vi "Save Lockin Metadata.vi"(8 "error in (no error)":errorcluster, 11 "Lockin Digitizer Driver in":refnum<class "Lockin Digitizer Driver.lvclass">) -> (0 "error out":errorcluster, 3 "Lockin Digitizer Driver out":refnum<class "Lockin Digitizer Driver.lvclass">)   [LabVIEW 2024, in "Lockin Digitizer Driver.lvclass"]
uses:
  Lockin Digitizer Driver.lvclass
  Pulse Driver.lvclass/Pulse Driver.ctl
  SoftwareLockin/Lockin Parameters.ctl
  Read tdms file.vi
  Write tdms file.vi
  Lockin Digitizer Driver.lvclass/Lockin Digitizer Driver.ctl
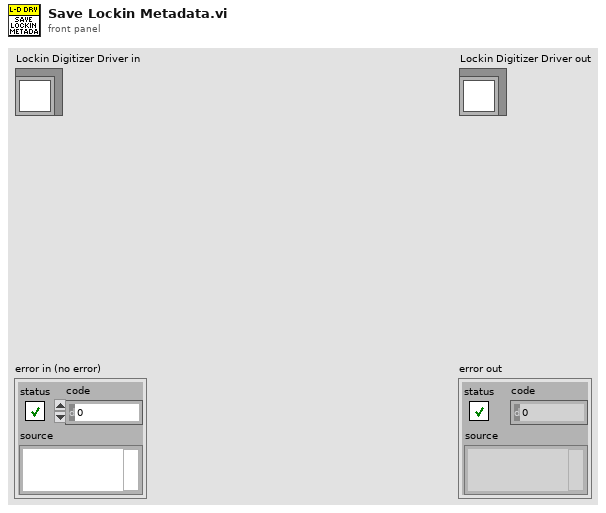
[diagram p1: front panel]
types:
  T1 = typedef "Lockin Digitizer Configuration.ctl" = cluster{"Post-trigger delay":dbl, "Post-trigger duration":dbl, "Rate":dbl, "Ranges":dbl[], "Re-name channels":string[], "Active channels":string, "External\nclock":bool, "Monitor time\nconstant":dbl, "Sync":bool, "Lock-in input channel phases":dbl[], "Output channels configuration":T2[]}
  T2 = typedef "Output Channel Configuration.ctl" = cluster{"Input channels":string, "Frequency":dbl, "Output amplitude":dbl, "Output channel number":i32}
  T3 = typedef "Lockin Parameters.ctl" = cluster{"Frequency":dbl, "Phase":dbl, "Syncronous":bool, "Points per sine wave":i32, "DDS":bool, "Frequency word":u32, "Phase word":u32, "DDS modulus":i64, "DDS clock":dbl}
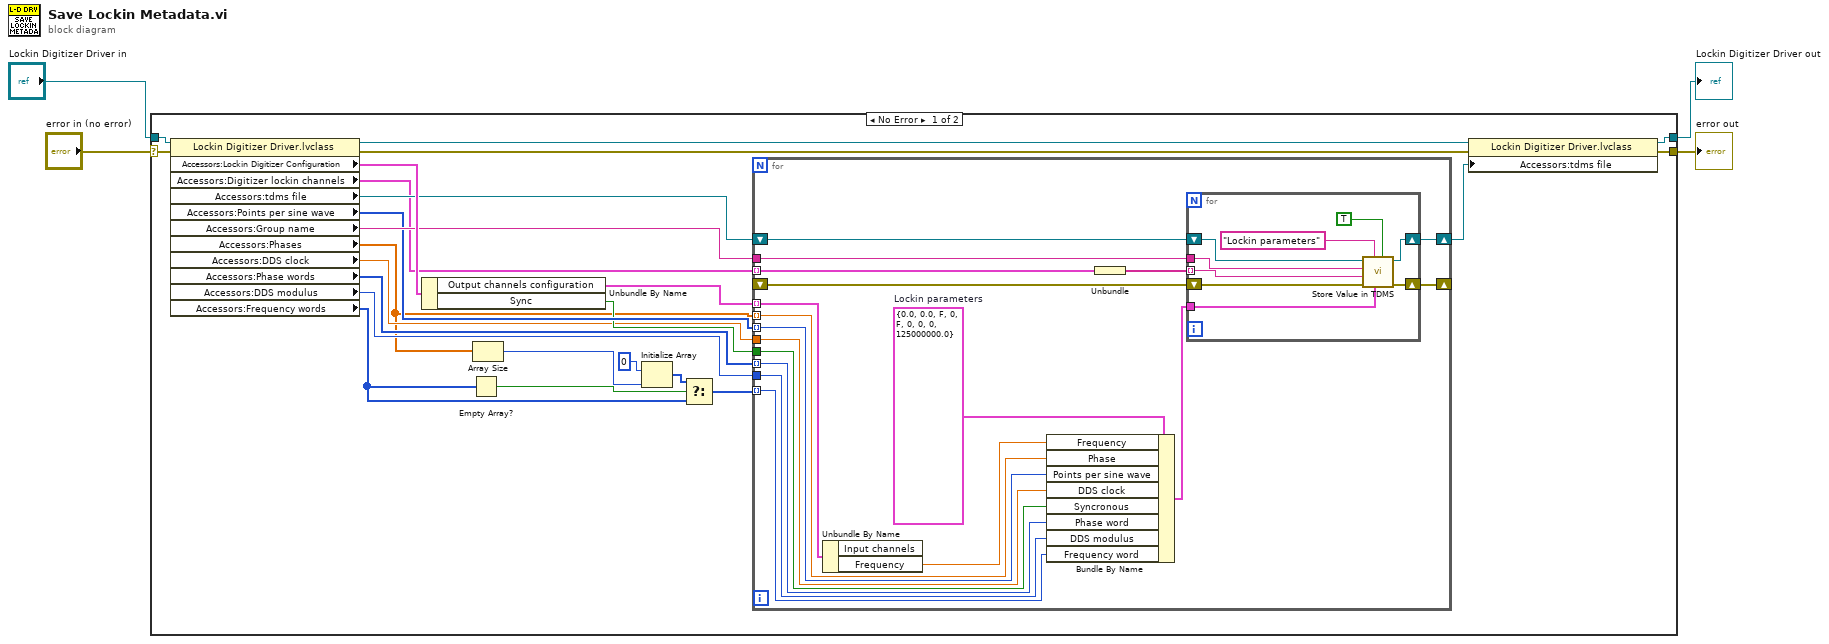
[diagram p0: block diagram]
diagram:
  n1 = case shown="No Error" "error in (no error)" {
    selector: "error in (no error)" -> [w28 w57]
    tunnel: [w22 w57] -> w3
    tunnel: [w20 w56] -> w1
    tunnel: "Lockin Digitizer Driver in" -> [w26 w56]
    frame No Error {
      n2 = property class="Lockin Digitizer Driver.lvclass"(reference=w26, error in=w28) -> (reference out=w21:refnum<class "Lockin Digitizer Driver.lvclass">, error out=w27:errorcluster, "Accessors:Lockin Digitizer Configuration"=w25:T1, "Accessors:Digitizer lockin channels"=w12:cluster{string[]}[], "Accessors:tdms file"=w18:refnum<k34>, "Accessors:Points per sine wave"=w17:i32[], "Accessors:Group name"=w23:string, "Accessors:Phases"=w10:dbl[], "Accessors:DDS clock"=w15:dbl, "Accessors:Phase words"=w14:u32[], "Accessors:DDS modulus"=w13:i64, "Accessors:Frequency words"=w6:u32[])
      n3 = Unbundle By Name(w25) -> ("Output channels configuration"=w24:T2[], "Sync"=w16:bool)
      n4 = Empty Array?(array=w6) -> (empty?=w11:bool)
      n5 = Array Size(array=w10) -> (size(s)=w8:i32)
      n6 = Initialize Array(u32 0 ("Numeric"), w8) -> (w7:u32[])
      n7 = Select(t=w7, s=w11, f=w6) -> (s? t:f=w5:u32[])
      n8 = for {
        tunnel: w24 -> [w45] mode=indexing
        tunnel: w12 -> [w39] mode=indexing
        tunnel: w15 -> [w44]
        shift-right: [w42] -> w19
        shift-left: w18 -> [w43]
        shift-right: [w40] -> _
        shift-left: _ -> [w41]
        tunnel: w23 -> [w37]
        tunnel: w16 -> [w35]
        tunnel: w17 -> [w34] mode=indexing
        tunnel: w10 -> [w33] mode=indexing
        tunnel: w14 -> [w32] mode=indexing
        tunnel: w13 -> [w31]
        tunnel: w5 -> [w29] mode=indexing
        w46 = T3 {"Frequency"=0.0, "Phase"=0.0, "Syncronous"=FALSE, "Points per sine wave"=0, "DDS"=FALSE, "Frequency word"=0, "Phase word"=0, "DDS modulus"=0, "DDS clock"=125000000.0}  # Lockin parameters
        n9 = Unbundle By Name(w45) -> ("Frequency"=w30:dbl)  [unwired: 1 out]
        n10 = Bundle By Name(cluster=w46, "Frequency"=w30, "Phase"=w33, "Points per sine wave"=w34, "DDS clock"=w44, "Syncronous"=w35, "Phase word"=w32, "DDS modulus"=w31, "Frequency word"=w29) -> (w36:T3)
        n11 = Unbundle(w39) -> (w38:string[])
        n12 = for {
          shift-right: [w54] -> w42
          shift-left: w43 -> [w55]
          shift-right: [w52] -> w40
          shift-left: w41 -> [w53]
          tunnel: w38 -> [w51] mode=indexing
          tunnel: w37 -> [w50]
          tunnel: w36 -> [w49]
          n13 = call "Store Value in TDMS.vi"("Replace name with prefix (FALSE = append)"=TRUE, "Value"=w49, "Prefix"="Lockin parameters", "Error In"=w53, "channel name"=w51, "group name"=w50, "tdms file"=w55) -> ("Error Out"=w52:errorcluster, "tdms file out"=w54:refnum<k34>)  [unwired: 1 in, 2 out]
        }
      }
      n14 = property class="Lockin Digitizer Driver.lvclass"(reference=w21, error in=w27, "Accessors:tdms file"=w19) -> (reference out=w20:refnum<class "Lockin Digitizer Driver.lvclass">, error out=w22:errorcluster)
    }
    frame Error {
    }
  }
  "error out" <- w3
  "Lockin Digitizer Driver out" <- w1
